vi "String List to Combo String.vi"(1 "find list":string[](array[string])) -> (0 "String":string)   [LabVIEW 2016, in "Controller UI.lvlib" / "Controller UI.lvclass"]
uses:
  <userlib>/Common Components/Controller UI/Controller UI.lvclass
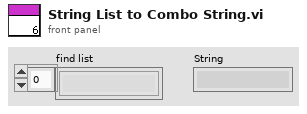
[diagram p1: front panel]
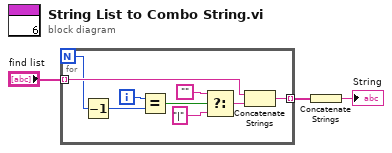
[diagram p0: block diagram]
diagram:
  n1 = for {
    N -> [w9]
    tunnel: "find list" -> [w12] mode=indexing
    tunnel: [w11] -> w2 mode=indexing
    i -> [w10]
    n2 = Decrement(x=w9) -> (x-1=w8:i32)
    n3 = Equal?(x=w10, y=w8) -> (x = y?=w7:bool)
    n4 = Select(t="", s=w7, f="|" ("string")) -> (s? t:f=w4:string)
    n5 = Concatenate Strings(w12, w4) -> (w11:string)
  }
  n6 = Concatenate Strings(w2) -> (→"String":string)
